vi "Stage Format JSON input.vi"(8 "error in (no error)":errorcluster, 11 "JSON string (in)":string) -> (0 "error out":errorcluster, 2 "ESC Internal Data Structure (with types)":T2={"Test_File"=path "", "Status"="Done", "RF_Center_Freq"=0.0, "RF_Gain"=0.0, "BB_Gain"=0.0, "Error 2"="", "file_max"=0, "file_index"=0}, 3 "Internal Vars":T1={"Test_File"="", "Status"="Done", "RF_Center_Freq"="0", "RF_Gain"="0", "BB_Gain"="0", "Error"="", "file_max"="0", "file_index"="0"})   [LabVIEW 2017]
uses:
  TypeDef/ESC Internal Data Structure (types).ctl
  TypeDef/ESC Internal Data Structure (string).ctl
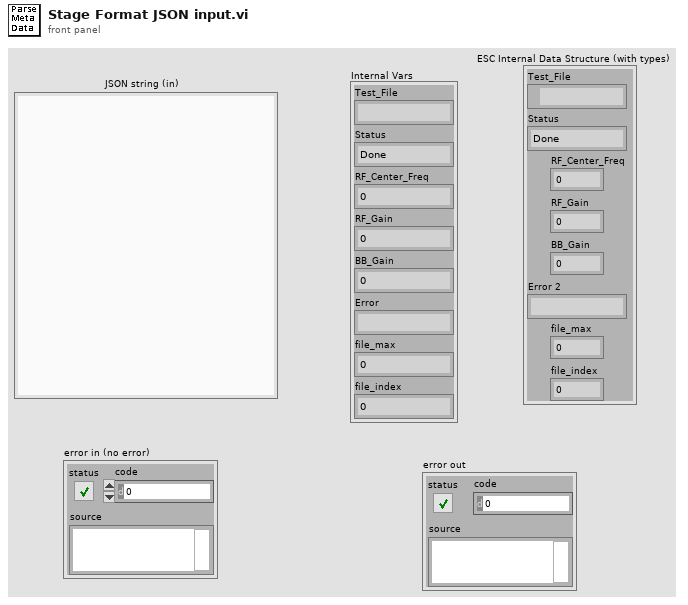
[diagram p1: front panel]
types:
  T1 = typedef "ESC Internal Data Structure (string).ctl" = cluster{"Test_File":string, "Status":string, "RF_Center_Freq":string, "RF_Gain":string, "BB_Gain":string, "Error":string, "file_max":string, "file_index":string}
  T2 = typedef "ESC Internal Data Structure (types).ctl" = cluster{"Test_File":path, "Status":string, "RF_Center_Freq":dbl, "RF_Gain":dbl, "BB_Gain":dbl, "Error 2":string, "file_max":u64, "file_index":u64}
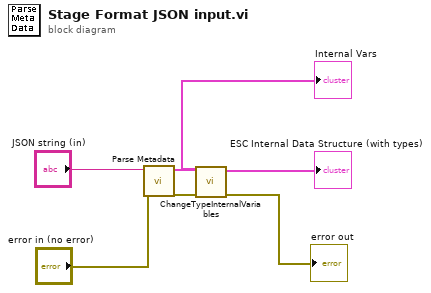
[diagram p0: block diagram]
diagram:
  n1 = call "Parse Metadata.vi"("error in"="error in (no error)", "JSON string (in)"="JSON string (in)") -> ("error out"=w5:errorcluster, "Internal Vars"=w6:T1)  [unwired: 8 in]
  "Internal Vars" <- w6
  n2 = call "ChangeTypeInternalVariables.vi"("error in"=w5, "ESC Internal Data Structure"=w6) -> ("error out"=→"error out":errorcluster, "ESC Internal Data Structure (with types)"=→"ESC Internal Data Structure (with types)":T2)  [unwired: 8 in]
